vi "DAQ_PW_SET_RANGE_UA_MA.vi"(8 "error in":errorcluster, 10 "Current Range":enum16{"Set uA Range ", "Set mA Range"}(ring), 11 "device name":tag="Dev4") -> (0 "error out":errorcluster)   [LabVIEW 2015]
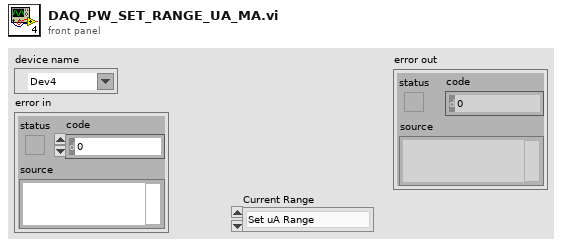
[diagram p1: front panel]
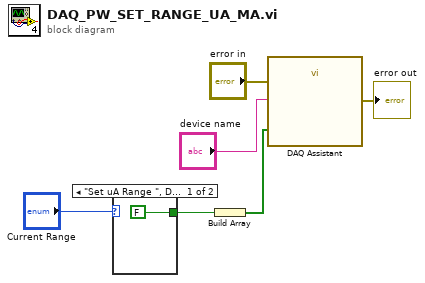
[diagram p0: block diagram]
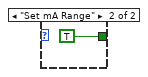
[diagram p2: hidden frame]
diagram:
  n1 = case shown="\"Set uA Range \", Default" "Current Range" {
    tunnel: [FALSE TRUE] -> w5
    frame "Set uA Range ", Default {
    }
    frame "Set mA Range" {
    }
  }
  n2 = Build Array(w5) -> (w4:bool[])
  n3 = call "DAQ Assistant"("data"=w4, "error in"="error in", "device name"="device name") -> ("error out"=→"error out":errorcluster)  [unwired: 15 in, 1 out]
